vi "Real-Time Main-Final_Local.vi"() -> ()   [LabVIEW 2024]
uses:
  <instrlib>/niScope/Controls/niScope trigger source.ctl
  <vilib>/Platform/TimedLoop/XDataNode/timing_clust.ctl
  <vilib>/Platform/TimedLoop/XDataNode/nitl_modes.ctl
  <vilib>/Platform/TimedLoop/XDataNode/wakeup.ctl
  <instrlib>/niScope/Configure/Trigger/niScope Configure Trigger Edge.vi
  <instrlib>/niScope/Acquire/Fetch/niScope Fetch WDT.vi
  <vilib>/Waveform/WDTOps.llb/WDT Get Waveform Time Array DBL.vi
  <vilib>/platform/TimedLoop/XDataNode/XDataNode.xnode
  <vilib>/Platform/TimedLoop/XDataNode/XDNodeRunTimeDep.lvlib
panel:
  in  "channels":string="0"
  in  "FileName":string
  out "Time_shift":dbl
  out "wfm":waveform(dbl)(graph)
  out "# of Chunks Fetched":i32
  out "# of Points Fetched":i32
  in  "stop":bool
  in  "Resource Name":refnum<k15>="Dev1" caption="Resource Name(s)"
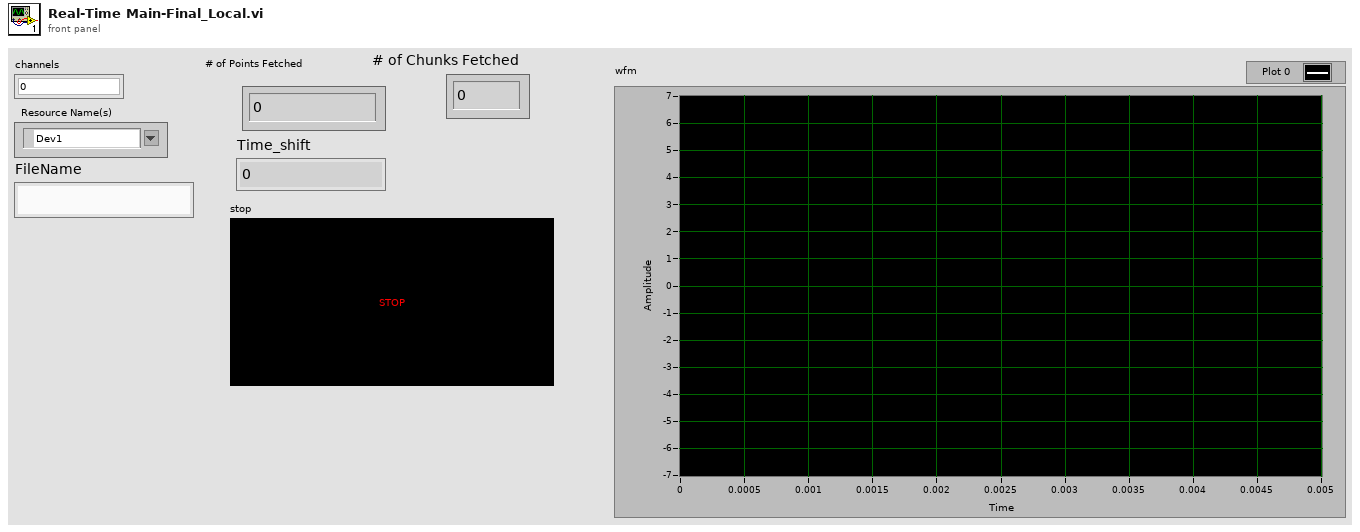
[diagram p1: front panel]
types:
  T1 = typedef "niScope trigger source.ctl" = string
  T2 = enum16{"open", "open or create", "create or replace", "create", "open (read-only)"}
  T3 = typedef "XDNodeRunTimeDep.lvlib/timing_clust.ctl" = cluster{"Expected End [f-1]":u64, "Actual End [f-1]":u64, "Finished Late? [f-1]":bool, "Expected End [i-1]":u64, "Actual End [i-1]":u64, "Finished Late? [i-1]":bool, "Expected Start [i]":u64, "Actual Start [i]":u64, "Expected Start [f]":u64, "Actual Start [f]":u64, "Source Name":string, "Structure Name":string, "Period":i64, "Deadline":i64, "Offset":i64, "Start":i64, "Priority":i32, "Timeout":i32, "Mode":T4, "Wakeup Reason":T5, "Error":errorcluster, "Source Type":string, "Secondary Source Type":string, "Global End Time":u64, "Global Start Time":u64, "Frame Duration":u64, "Iteration Duration":u64, "Assigned CPU":i32, "I/O Scan Engine Mode":u32}
  T4 = typedef "XDNodeRunTimeDep.lvlib/nitl_modes.ctl" = enum32{"No Change", "Process missed periods, maintain original phase", "Discard missed periods, maintain original phase", "Process missed periods, ignore original phase", "Discard missed periods, ignore original phase"}
  T5 = typedef "XDNodeRunTimeDep.lvlib/wakeup.ctl" = enum32{"Normal", "Aborted", "Asynchronous wakeup", "Timing source error", "Timed loop error", "Timeout"}
  T6 = cluster{"actualSamples":i32, "absoluteInitialX":dbl, "relativeInitialX":dbl, "xIncrement":dbl, "offset":dbl, "gain":dbl, "reserved1":dbl, "reserved2":dbl}
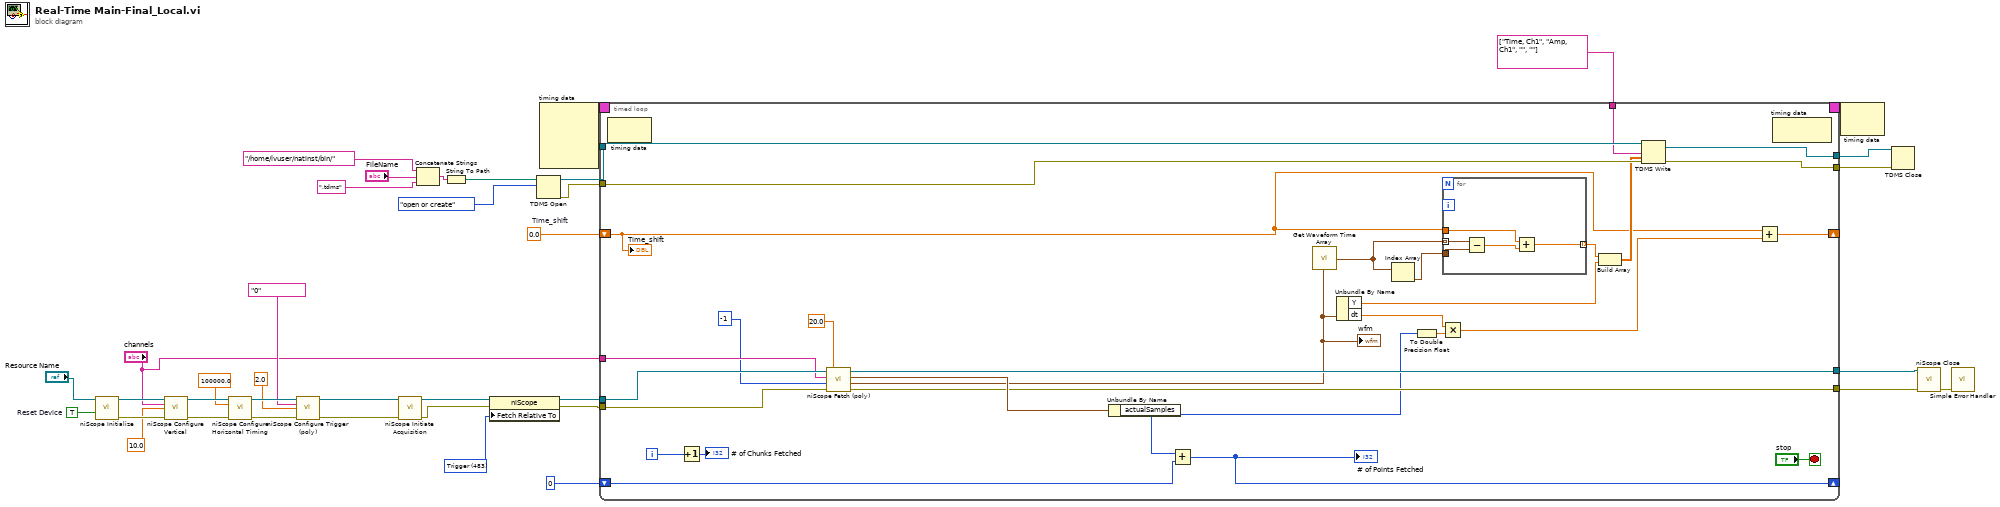
[diagram p0: block diagram]
diagram:
  w1 = 483 items=["Start"=482, "Trigger"=483, "Pretrigger"=477, "Now"=481, "Read Pointer"=388] ("Fetch:Fetch Relative To")
  w24 = 0.0  # Time_shift
  w36 = TRUE  # Reset Device
  n1 = call <instrlib>:"niScope Initialize.vi"("resource name"="Resource Name", "reset device"=w36) -> ("instrument handle"=w17:refnum<k15>, "error out"=w16:errorcluster)  [unwired: 12 in]
  n2 = call <instrlib>:"niScope Configure Vertical.vi"("instrument handle"=w17, "channels"="channels", "vertical range"=10.0, "error in"=w16) -> ("instrument handle out"=w14:refnum<k15>, "error out"=w18:errorcluster)  [unwired: 10 in]
  n3 = call <instrlib>:"niScope Configure Horizontal Timing.vi"("instrument handle"=w14, "min sample rate"=100000.0, "error in"=w18) -> ("instrument handle out"=w12:refnum<k15>, "error out"=w11:errorcluster)  [unwired: 11 in]
  n4 = call-poly <instrlib>:"niScope Configure Trigger (poly).vi"("instrument handle"=w12, "trigger source"=T1 "0", "trigger level"=2.0, "error in"=w11) -> ("instrument handle out"=w9:refnum<k15>, "error out"=w8:errorcluster)  [unwired: 10 in]
  n5 = call <instrlib>:"niScope Initiate Acquisition.vi"("instrument handle"=w9, "error in"=w8) -> ("instrument handle out"=w7:refnum<k15>, "error out"=w6:errorcluster)  [unwired: 12 in]
  n6 = Concatenate Strings("/home/lvuser/natinst/bin/" ("string"), "FileName", ".tdms" ("string")) -> (w23:string)
  n7 = String To Path(string=w23) -> (path=w21:path)
  n8 = property class="niScope"(reference=w7, error in=w6, "Fetch Relative To"=w1) -> (reference out=w5:refnum<k15>, error out=w4:errorcluster)
  n9 = TDMS Open(10:T2."open or create" ("operation (0:open)"), 11:w21) -> (0:w27:errorcluster, 3:w26:refnum<k34>)  [unwired: 5 in]
  n10 = node-c288() -> (w38:T3)  [unwired: 4 in]
  n11 = timed-loop {
    timing: w38 -> [_]
    timing-out: [_] -> w37
    tunnel: [w67] -> w34
    shift-right: [w65] -> _
    shift-left: 0 -> [w66]
    tunnel: [w55] -> w31
    tunnel: w26 -> [w60]
    tunnel: w27 -> [w59]
    tunnel: [w58] -> w29
    tunnel: [w57] -> w28
    tunnel: string[] ["Time, Ch1", "Amp, Ch1", "", ""] ("channel name(s) in (Untitled)") -> [w56]
    shift-right: [w47] -> _
    shift-left: w24 -> [w46]
    tunnel: w5 -> [w42]
    tunnel: w4 -> [w41]
    tunnel: "channels" -> [w40]
    i -> [w64]
    stop <- "stop" stop-if-true
    n12 = node-c288() -> ()  [unwired: 1 in, 1 out]
    n13 = Increment(x=w64) -> (x+1=→"# of Chunks Fetched":i32)
    n14 = call-poly <instrlib>:"niScope Fetch (poly).vi"("timeout"=20.0, "error in"=w41, "numSamples"=-1, "channels"=w40, "instrument handle"=w42) -> ("error out"=w55:errorcluster, "wfm"=w49:waveform(dbl), "wfm info"=w63:T6, "instrument handle out"=w67:refnum<k15>)  [unwired: 3 in]
    "wfm" <- w49
    n15 = Unbundle By Name(w63) -> ("actualSamples"=w45:i32)
    n16 = Add(x=w45, y=w66) -> (x+y=w65:i32)
    "# of Points Fetched" <- w65
    n17 = call-poly <vilib>:"Get Waveform Time Array.vi"("waveform in"=w49) -> ("X array"=w50:timestamp[])  [unwired: 9 in, 1 out]
    n18 = Unbundle By Name(w49) -> ("Y"=w54:dbl[], "dt"=w44:dbl)
    n19 = Index Array(array=w50) -> (element=w51:timestamp)  [unwired: 1 in]
    n20 = To Double Precision Float(number=w45) -> (double precision float=w48:dbl)
    n21 = Multiply(x=w44, y=w48) -> (x*y=w43:dbl)
    n22 = for {
      tunnel: [w71] -> w52 mode=indexing
      tunnel: w51 -> [w73]
      tunnel: w50 -> [w72] mode=indexing
      tunnel: w46 -> [w69]
      n23 = Subtract(x=w72, y=w73) -> (x-y=w70:dbl)
      n24 = Add(x=w69, y=w70) -> (x+y=w71:dbl)
    }
    n25 = Build Array(w52, w54) -> (w53:dbl[][])
    n26 = TDMS Write(0:w60, 7:w56, 9:w53, 11:w59) -> (4:w58:refnum<k34>, 15:w57:errorcluster)  [unwired: 2 in, 2 out]
    n27 = Add(x=w46, y=w43) -> (x+y=w47:dbl)
    n28 = node-c288() -> ()  [unwired: 1 in, 1 out]
    "Time_shift" <- w46
  }
  n29 = node-c288(w37) -> ()  [unwired: 1 out]
  n30 = TDMS Close(8:w28, 11:w29) -> ()  [unwired: 2 out]
  n31 = call <instrlib>:"niScope Close.vi"("instrument handle"=w34, "error in"=w31) -> ("error out"=w32:errorcluster)  [unwired: 13 in]
  n32 = call <vilib>:"Simple Error Handler.vi"("error in (no error)"=w32) -> ()  [unwired: 4 in, 5 out]
